vi "Helper SubVI - Sine Curve Fitting Core.vi"(7 "signal in":waveform(dbl), 11 "ADT paras":T1(array[cluster])) -> (1 "Frequencies":dbl[](array[numeric]) format="%.2f", 2 "Amplitudes":dbl[](array[numeric]) format="%.2f", 3 "signal out":waveform(dbl), 4 "Offset":dbl[](array[numeric]) format="%.2f", 5 "Phases":dbl[](array[numeric]) format="%.2f")   [LabVIEW 2023]
doc: "Computes the parameters of sine waves."
uses:
  <vilib>/Waveform/WDTOps.llb/WDT Number of Waveform Samples DBL.vi
  <vilib>/Analysis/NI_AALBase.lvlib
  <vilib>/Analysis/NI_AALPro.lvlib
panel:
  in  "empty":waveform(dbl)={"t0"=timestamp(0 s since 1904-01-01), "dt"=0.0, "Y"=[]}
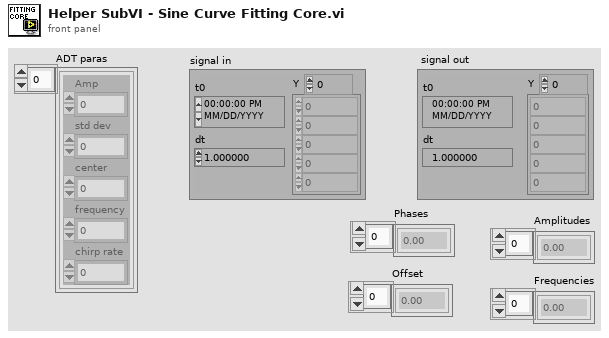
[diagram p1: front panel]
types:
  T1 = cluster{"Amp":cdb, "std dev":dbl, "center":dbl, "frequency":dbl, "chirp rate":dbl}[]
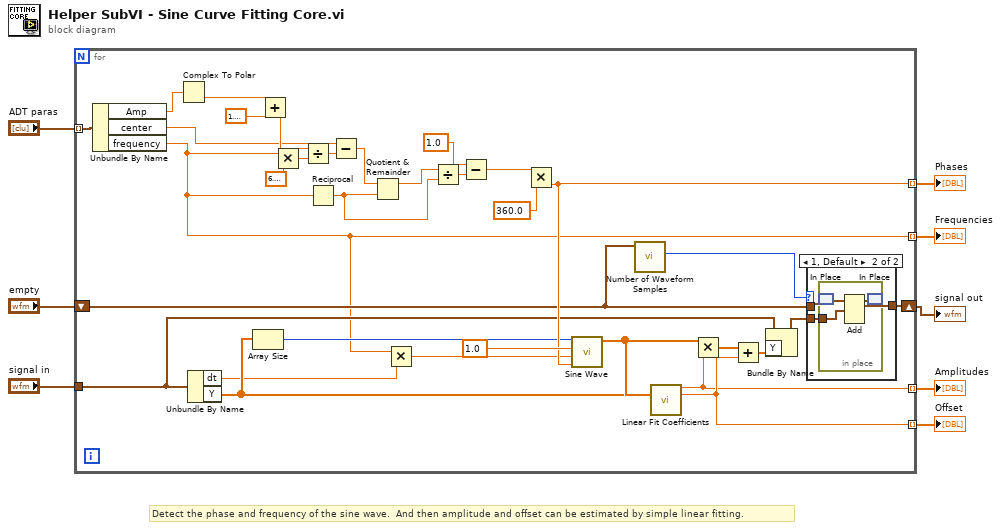
[diagram p0: block diagram]
diagram:
  # "Detect the phase and frequency of the sine wave.  And then amplitude and offset can be estimated by simple linear fitting."
  n1 = for {
    tunnel: [w39] -> w8 mode=indexing
    tunnel: [w37] -> w7 mode=indexing
    tunnel: [w24] -> w6 mode=indexing
    tunnel: "signal in" -> [w20]
    tunnel: [w9] -> w4 mode=indexing
    shift-right: [w15] -> w3
    shift-left: "empty" -> [w14]
    tunnel: "ADT paras" -> [w12] mode=indexing
    n2 = Unbundle By Name(w12) -> ("Amp"=w11:cdb, "center"=w10:dbl, "frequency"=w9:dbl)
    n3 = Complex To Polar(r * e^(i*theta)=w11) -> (theta=w17:dbl)  [unwired: 1 out]
    n4 = Unbundle By Name(w20) -> ("dt"=w18:dbl, "Y"=w23:dbl[])
    n5 = Array Size(array=w23) -> (size(s)=w22:i32)
    n6 = Add(x=w17, y=1.5707963267948966 ("Pi Divided By 2")) -> (x+y=w30:dbl)
    n7 = Multiply(x=w9, y=6.283185307179586 ("Pi Multiplied By 2")) -> (x*y=w40:dbl)
    n8 = Divide(x=w30, y=w40) -> (x/y=w29:dbl)
    n9 = Reciprocal(x=w9) -> (1/x=w26:dbl)
    n10 = Subtract(x=w10, y=w29) -> (x-y=w33:dbl)
    n11 = Quotient & Remainder(x=w33, y=w26) -> (x-y*floor(x/y)=w35:dbl)  [unwired: 1 out]
    n12 = Multiply(x=w9, y=w18) -> (x*y=w19:dbl)
    n13 = Divide(x=w35, y=w26) -> (x/y=w32:dbl)
    n14 = Subtract(x=1.0, y=w32) -> (x-y=w28:dbl)
    n15 = Multiply(x=w28, y=360.0) -> (x*y=w24:dbl)
    n16 = call <vilib>:"Sine Wave.vi"("samples"=w22, "amplitude"=1.0, "frequency"=w19, "phase in"=w24) -> ("sine wave"=w36:dbl[])  [unwired: 1 in, 2 out]
    n17 = call-poly <vilib>:"Number of Waveform Samples.vi"("waveform in"=w14) -> ("number of samples"=w13:i32)  [unwired: 1 in, 9 out]
    n18 = call <vilib>:"Linear Fit Coefficients.vi"("Y"=w23, "X"=w36) -> ("slope"=w37:dbl, "intercept"=w39:dbl)  [unwired: 3 in, 9 out]
    n19 = Multiply(x=w36, y=w37) -> (x*y=w38:dbl[])
    n20 = Add(x=w38, y=w39) -> (x+y=w21:dbl[])
    n21 = Bundle By Name(cluster=w20, "Y"=w21) -> (w16:waveform(dbl))
    n22 = case shown="1, Default" w13 {
      tunnel: w16 -> [w42 w45]
      tunnel: [w42 w44] -> w15
      tunnel: w14 -> [_ w43]
      frame 0 {
      }
      frame 1, Default {
        n23 = in-place {
          in-place-border: w45 -> [w48]
          n24 = in-place-match #1(w43) -> (w46:waveform(dbl))
          n25 = Add(1:w48, 2:w46) -> (0:w47:waveform(dbl))  [unwired: 1 in, 1 out]
          n26 = in-place-match #1(w47) -> (w44:waveform(dbl))
        }
      }
    }
  }
  "Frequencies" <- w4
  "Offset" <- w8
  "signal out" <- w3
  "Amplitudes" <- w7
  "Phases" <- w6
